vi "sine_add_FFT.vi"() -> ()   [LabVIEW 2016]
uses:
  <vilib>/Analysis/2dsp.llb/Power Spectrum (DBL).vi
  <vilib>/Analysis/2dsp.llb/Real FFT.vi
  <vilib>/Analysis/NI_AALPro.lvlib
panel:
  out "Waveform Graph 6":dynamicdata(graph)
  out "Waveform Graph 5":dynamicdata(graph)
  out "Boolean":bool
  out "x*y":dbl
  out "Waveform Graph 4":dbl[](graph)
  out "FFT {X}":cdb[](array[numeric])
  out "Numeric 2":dbl
  out "Minimum":dbl
  out "Maximum":dbl
  out "Waveform Graph 2":dynamicdata(graph)
  out "Waveform Graph 3":dynamicdata(graph)
  in  "stop":bool
  out "Waveform Graph":dynamicdata(graph)
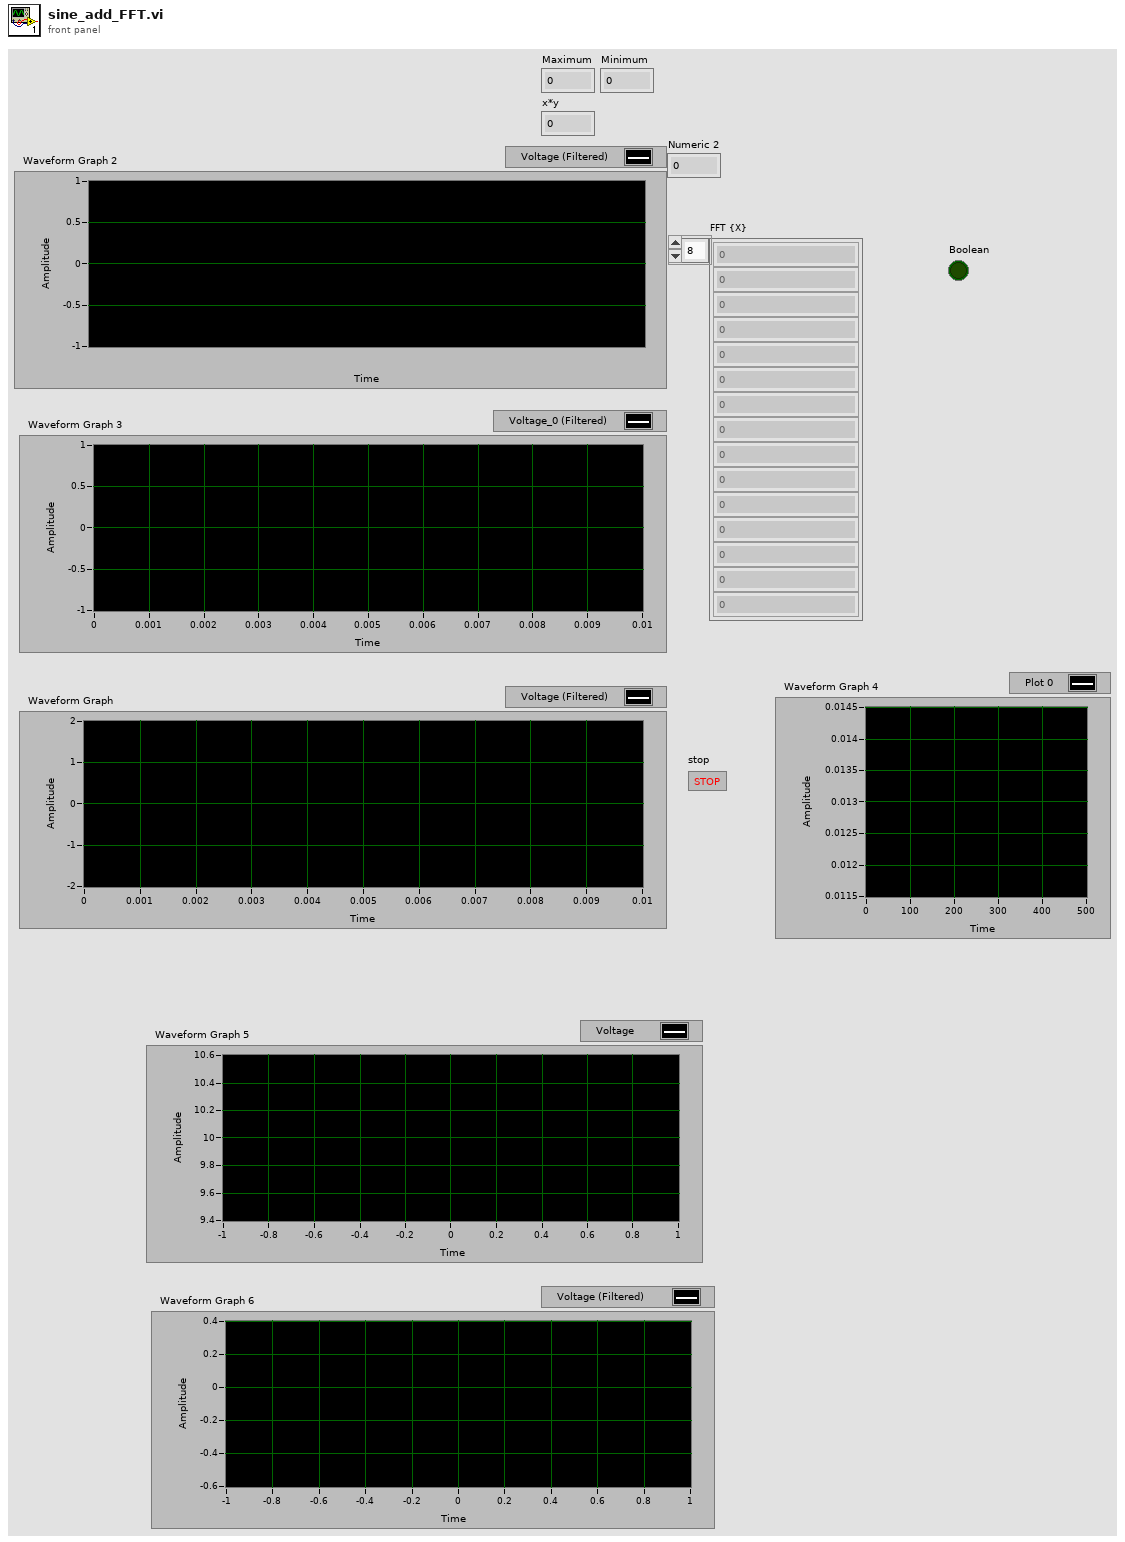
[diagram p1: front panel]
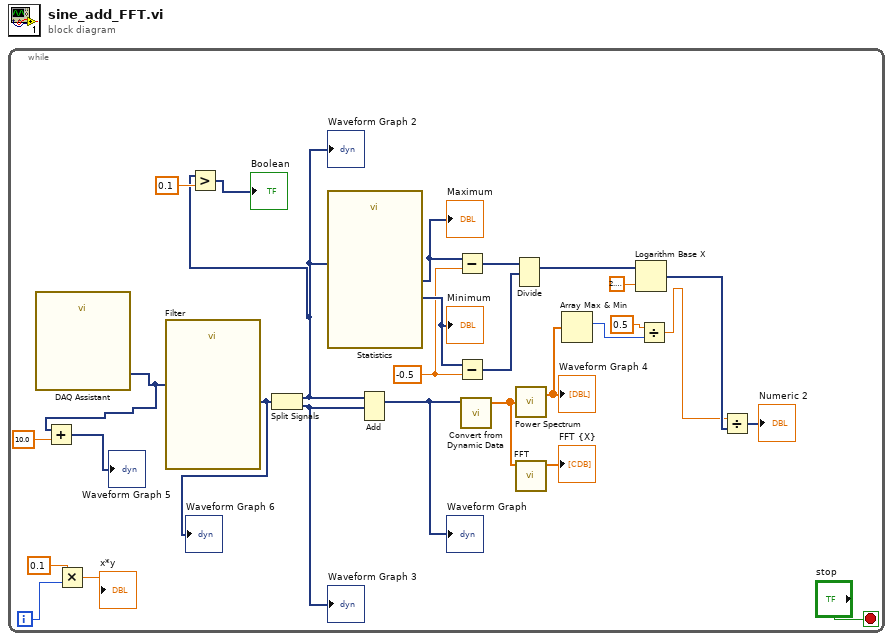
[diagram p0: block diagram]
diagram:
  n1 = while {
    i -> [w11]
    stop <- "stop" stop-if-true
    w24 = -0.5
    n2 = call "DAQ Assistant"() -> ("data"=w2:dynamicdata)  [unwired: 16 in, 3 out]
    n3 = Add(x=w2, y=10.0) -> (x+y=→"Waveform Graph 5":dynamicdata)
    n4 = Multiply(x=0.1, y=w11) -> (x*y=→"x*y":dbl)
    n5 = call "Filter"("Signal"=w2) -> ("Filtered Signal"=w1:dynamicdata)  [unwired: 9 in, 1 out]
    "Waveform Graph 6" <- w1
    n6 = Split Signals(w1) -> (w5:dynamicdata, w6:dynamicdata)  [unwired: 2 in]
    "Waveform Graph 3" <- w6
    "Waveform Graph 2" <- w5
    n7 = Greater?(x=w5, y=0.1) -> (0:→"Boolean":dynamicdata)
    n8 = call "Statistics"("Signals"=w5) -> ("Minimum"=w25:dynamicdata, "Maximum"=w26:dynamicdata)  [unwired: 22 in, 3 out]
    "Maximum" <- w26
    "Minimum" <- w25
    n9 = Add(1:w6, 2:w5) -> (0:w27:dynamicdata)  [unwired: 1 in, 1 out]
    "Waveform Graph" <- w27
    n10 = Subtract(x=w26, y=w24) -> (x-y=w23:dynamicdata)
    n11 = Subtract(x=w25, y=w24) -> (x-y=w22:dynamicdata)
    n12 = call "Convert from Dynamic Data"("Dynamic Data Type"=w27) -> ("Array"=w18:dbl[])  [unwired: 3 in]
    n13 = Divide(1:w22, 2:w23) -> (0:w21:dynamicdata)  [unwired: 1 in, 1 out]
    n14 = call-poly <vilib>:"Power Spectrum.vi"("X"=w18) -> ("Power Spectrum"=w17:dbl[])  [unwired: 1 out]
    "Waveform Graph 4" <- w17
    n15 = call-poly <vilib>:"FFT.vi"("X"=w18) -> ("FFT {X}"=→"FFT {X}":cdb[])  [unwired: 9 in, 1 out]
    n16 = Array Max & Min(array=w17) -> (max index (indices)=w16:i32)  [unwired: 3 out]
    n17 = Logarithm Base X(1:2.718281828459045, 2:w21) -> (0:w13:dynamicdata)
    n18 = Divide(x=0.5, y=w16) -> (x/y=w12:dbl)
    n19 = Divide(x=w12, y=w13) -> (x/y=→"Numeric 2":dynamicdata)
  }
